vi "update_clock.vi"(8 "update command in":bool, 9 "update reset counter in":bool, 10 "data sending counter (#bytes) in":u32, 11 "reset counter in":u8) -> (1 "update reset counter out":bool, 2 "data sending counter (#bytes) out":u32, 3 "reset counter out":u8)   [LabVIEW 2010]
uses:
  <vilib>/eio/EIONode/EIONode.xnode
  <vilib>/rvi/eio/nirviEIOImplementation/nirviEIOImplementation.xnode
  <vilib>/rvi/eio/common/nirviEmuClasses.ctl
  <vilib>/rvi/eio/common/nirviEmuTemplateMethod_noerrors.vi
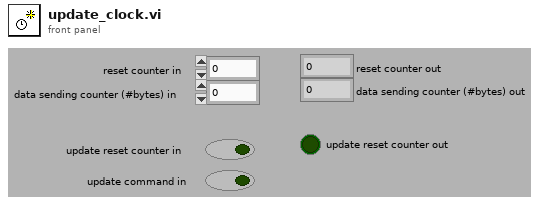
[diagram p1: front panel]
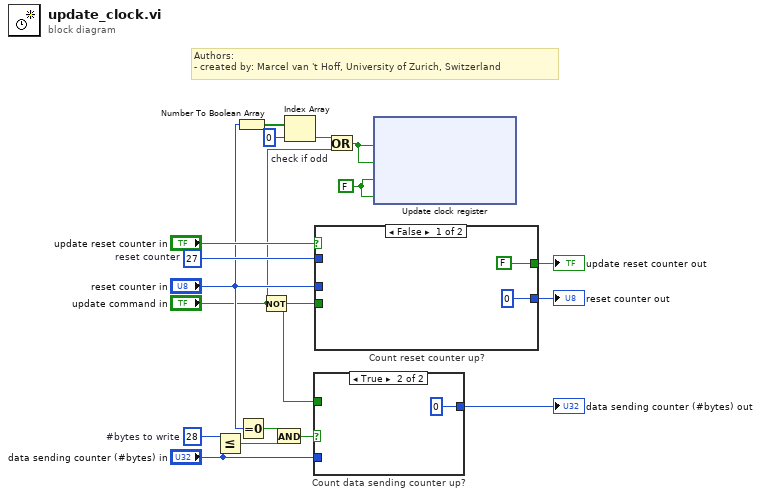
[diagram p0: block diagram]
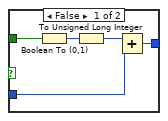
[diagram p2: hidden frame]
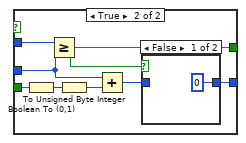
[diagram p3: hidden frame]
diagram:
  w12 = u8 27  # reset counter
  w16 = u32 28  # #bytes to write
  w18 = FALSE ("start acquisition")
  # "Authors: \n- created by: Marcel van 't Hoff, University of Zurich, Switzerland"
  n1 = Less Or Equal?(x=w16, y="data sending counter (#bytes) in") -> (x <= y?=w15:bool)
  n2 = Number To Boolean Array(number="reset counter in") -> (Boolean array=w5:bool[])
  n3 = Equal To 0?(x="reset counter in") -> (x = 0?=w14:bool)
  n4 = Not(x="update command in") -> (.not. x?=w10:bool)
  n5 = And(x=w14, y=w15) -> (x .and. y?=w7:bool)
  n6 = Index Array "check if odd"(array=w5, index=0) -> (element=w3:bool)
  n7 = case "Count data sending counter up?" shown="True" w7 {
    tunnel: "data sending counter (#bytes) in" -> [w23 _]
    tunnel: [w22 u32 0] -> w9
    tunnel: w10 -> [w19 _]
    frame False {
      n8 = Boolean To (0,1)(Boolean=w19) -> (0, 1=w21:i16)
      n9 = To Unsigned Long Integer(number=w21) -> (unsigned 32bit integer=w20:u32)
      n10 = Add(x=w20, y=w23) -> (x+y=w22:u32)
    }
    frame True {
    }
  }
  "data sending counter (#bytes) out" <- w9
  n11 = case "Count reset counter up?" shown="False" "update reset counter in" {
    tunnel: [u8 0 w29] -> w17
    tunnel: "reset counter in" -> [_ w31]
    tunnel: w10 -> [_ w33]
    tunnel: w12 -> [_ w30]
    tunnel: [FALSE w27] -> w11
    frame False {
    }
    frame True {
      n12 = Boolean To (0,1)(Boolean=w33) -> (0, 1=w34:i16)
      n13 = Greater Or Equal?(x=w30, y=w31) -> (x >= y?=w27:bool)
      n14 = To Unsigned Byte Integer(number=w34) -> (unsigned 8bit integer=w32:u8)
      n15 = Add(x=w31, y=w32) -> (x+y=w28:u8)
      n16 = case shown="False" w27 {
        tunnel: [u8 0 w36] -> w29
        tunnel: w28 -> [_ w36]
        frame False {
        }
        frame True {
        }
      }
    }
  }
  "reset counter out" <- w17
  "update reset counter out" <- w11
  n17 = Or(x=w3, y="update command in") -> (x .or. y?=w2:bool)
  n18 = xnode "Update clock register"("Connector3/DIO31"=w2, "Connector3/DIO29"=w2, "Connector3/DIO30"=w18, "Connector3/DIO28"=w18) -> ()  [unwired: 4 in, 4 out]
